vi "UpdateQueue.vi"(8 "error in (no error)":errorcluster, 9 "Queue Process":T1, 11 "ParameterConf in":refnum<class "ParameterConf.lvclass">) -> (0 "error out":errorcluster, 3 "ParameterConf out":refnum<class "ParameterConf.lvclass">)   [LabVIEW 2017, in "ParameterConf.lvclass"]
uses:
  ParameterConf.lvclass
  controls/QueueControl.ctl
  controls/CommandQueue.ctl
  ParameterConf.lvclass/ParameterConf.ctl
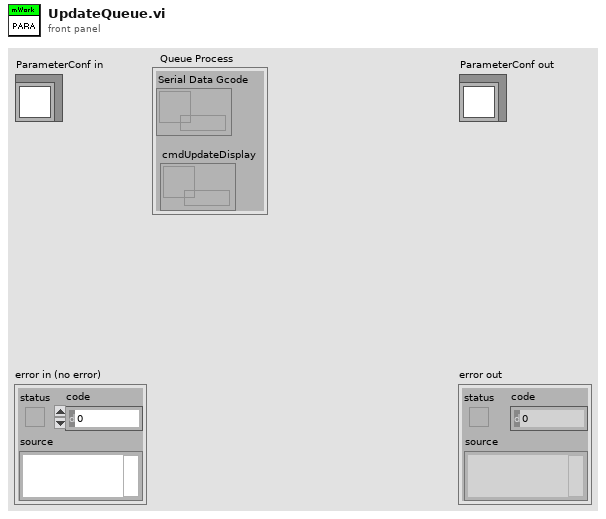
[diagram p1: front panel]
types:
  T1 = typedef "QueueControl.ctl" = cluster{"Serial Data Gcode":refnum<queue>, "cmdUpdateDisplay":refnum<queue>}
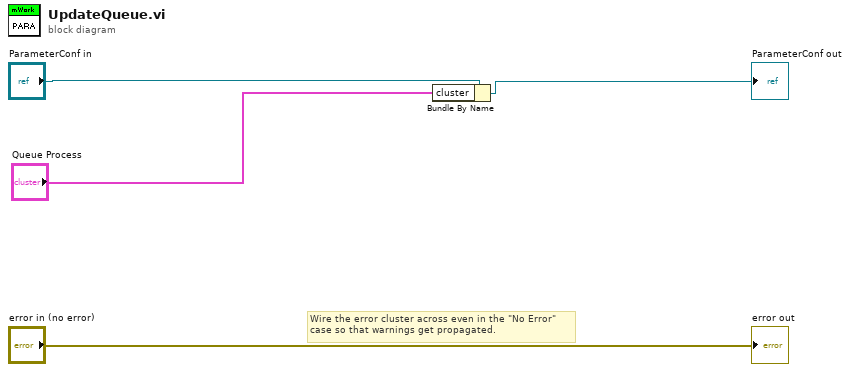
[diagram p0: block diagram]
diagram:
  # "Wire the error cluster across even in the \"No Error\"\ncase so that warnings get propagated."
  n1 = Bundle By Name(cluster="ParameterConf in", "cluster"="Queue Process") -> (→"ParameterConf out":refnum<class "ParameterConf.lvclass">)
  "error out" <- "error in (no error)"
